vi "OCV Histogram gRPC.vi"() -> (1 "mean values of channels":dbl[](array[numeric]), 2 "std dev":dbl, 3 "range":dbl)   [LabVIEW 2019] (continued)
"battery22voltage"=0.0, "battery23voltage"=0.0, "battery24voltage"=0.0, "ErrorOutData"={"ErrorCode"=0, "ErrorMessage"=""}}, {"battery1voltage"=3.4816399, "battery2voltage"=3.483045, "battery3voltage"=3.4783711, "battery4voltage"=3.482368, "battery5voltage"=3.4843976, "battery6voltage"=0.0, "battery7voltage"=0.0, "battery8voltage"=0.0, "battery9voltage"=0.0, "battery10voltage"=0.0, "battery11voltage"=0.0, "battery12voltage"=0.0, "battery13voltage"=0.0, "battery14voltage"=0.0, "battery15voltage"=0.0, "battery16voltage"=0.0, "battery17voltage"=0.0, "battery18voltage"=0.0, "battery19voltage"=0.0, "battery20voltage"=0.0, "battery21voltage"=0.0, "battery22voltage"=0.0, "battery23voltage"=0.0, "battery24voltage"=0.0, "ErrorOutData"={"ErrorCode"=0, "ErrorMessage"=""}}, {"battery1voltage"=3.4816442, "battery2voltage"=3.4830372, "battery3voltage"=3.4783738, "battery4voltage"=3.482372, "battery5voltage"=3.4844053, "battery6voltage"=0.0, "battery7voltage"=0.0, "battery8voltage"=0.0, "battery9voltage"=0.0, "battery10voltage"=0.0, "battery11voltage"=0.0, "battery12voltage"=0.0, "battery13voltage"=0.0, "battery14voltage"=0.0, "battery15voltage"=0.0, "battery16voltage"=0.0, "battery17voltage"=0.0, "battery18voltage"=0.0, "battery19voltage"=0.0, "battery20voltage"=0.0, "battery21voltage"=0.0, "battery22voltage"=0.0, "battery23voltage"=0.0, "battery24voltage"=0.0, "ErrorOutData"={"ErrorCode"=0, "ErrorMessage"=""}}, {"battery1voltage"=3.4816413, "battery2voltage"=3.4830437, "battery3voltage"=3.4783747, "battery4voltage"=3.482368, "battery5voltage"=3.4843984, "battery6voltage"=0.0, "battery7voltage"=0.0, "battery8voltage"=0.0, "battery9voltage"=0.0, "battery10voltage"=0.0, "battery11voltage"=0.0, "battery12voltage"=0.0, "battery13voltage"=0.0, "battery14voltage"=0.0, "battery15voltage"=0.0, "battery16voltage"=0.0, "battery17voltage"=0.0, "battery18voltage"=0.0, "battery19voltage"=0.0, "battery20voltage"=0.0, "battery21voltage"=0.0, "battery22voltage"=0.0, "battery23voltage"=0.0, "battery24voltage"=0.0, "ErrorOutData"={"ErrorCode"=0, "ErrorMessage"=""}}, {"battery1voltage"=3.481636, "battery2voltage"=3.4830418, "battery3voltage"=3.4783738, "battery4voltage"=3.482369, "battery5voltage"=3.4844093, "battery6voltage"=0.0, "battery7voltage"=0.0, "battery8voltage"=0.0, "battery9voltage"=0.0, "battery10voltage"=0.0, "battery11voltage"=0.0, "battery12voltage"=0.0, "battery13voltage"=0.0, "battery14voltage"=0.0, "battery15voltage"=0.0, "battery16voltage"=0.0, "battery17voltage"=0.0, "battery18voltage"=0.0, "battery19voltage"=0.0, "battery20voltage"=0.0, "battery21voltage"=0.0, "battery22voltage"=0.0, "battery23voltage"=0.0, "battery24voltage"=0.0, "ErrorOutData"={"ErrorCode"=0, "ErrorMessage"=""}}, {"battery1voltage"=3.4816372, "battery2voltage"=3.4830408, "battery3voltage"=3.4783714, "battery4voltage"=3.4823658, "battery5voltage"=3.4844065, "battery6voltage"=0.0, "battery7voltage"=0.0, "battery8voltage"=0.0, "battery9voltage"=0.0, "battery10voltage"=0.0, "battery11voltage"=0.0, "battery12voltage"=0.0, "battery13voltage"=0.0, "battery14voltage"=0.0, "battery15voltage"=0.0, "battery16voltage"=0.0, "battery17voltage"=0.0, "battery18voltage"=0.0, "battery19voltage"=0.0, "battery20voltage"=0.0, "battery21voltage"=0.0, "battery22voltage"=0.0, "battery23voltage"=0.0, "battery24voltage"=0.0, "ErrorOutData"={"ErrorCode"=0, "ErrorMessage"=""}}, {"battery1voltage"=3.4816327, "battery2voltage"=3.4830406, "battery3voltage"=3.47837, "battery4voltage"=3.48237, "battery5voltage"=3.4844074, "battery6voltage"=0.0, "battery7voltage"=0.0, "battery8voltage"=0.0, "battery9voltage"=0.0, "battery10voltage"=0.0, "battery11voltage"=0.0, "battery12voltage"=0.0, "battery13voltage"=0.0, "battery14voltage"=0.0, "battery15voltage"=0.0, "battery16voltage"=0.0, "battery17voltage"=0.0, "battery18voltage"=0.0, "battery19voltage"=0.0, "battery20voltage"=0.0, "battery21voltage"=0.0, "battery22voltage"=0.0, "battery23voltage"=0.0, "battery24voltage"=0.0, "ErrorOutData"={"ErrorCode"=0, "ErrorMessage"=""}}, {"battery1voltage"=3.4816341, "battery2voltage"=3.4830384, "battery3voltage"=3.4783652, "battery4voltage"=3.4823718, "battery5voltage"=3.4844053, "battery6voltage"=0.0, "battery7voltage"=0.0, "battery8voltage"=0.0, "battery9voltage"=0.0, "battery10voltage"=0.0, "battery11voltage"=0.0, "battery12voltage"=0.0, "battery13voltage"=0.0, "battery14voltage"=0.0, "battery15voltage"=0.0, "battery16voltage"=0.0, "battery17voltage"=0.0, "battery18voltage"=0.0, "battery19voltage"=0.0, "battery20voltage"=0.0, "battery21voltage"=0.0, "battery22voltage"=0.0, "battery23voltage"=0.0, "battery24voltage"=0.0, "ErrorOutData"={"ErrorCode"=0, "ErrorMessage"=""}}, {"battery1voltage"=3.4816403, "battery2voltage"=3.4830394, "battery3voltage"=3.4783738, "battery4voltage"=3.482369, "battery5voltage"=3.4843953, "battery6voltage"=0.0, "battery7voltage"=0.0, "battery8voltage"=0.0, "battery9voltage"=0.0, "battery10voltage"=0.0, "battery11voltage"=0.0, "battery12voltage"=0.0, "battery13voltage"=0.0, "battery14voltage"=0.0, "battery15voltage"=0.0, "battery16voltage"=0.0, "battery17voltage"=0.0, "battery18voltage"=0.0, "battery19voltage"=0.0, "battery20voltage"=0.0, "battery21voltage"=0.0, "battery22voltage"=0.0, "battery23voltage"=0.0, "battery24voltage"=0.0, "ErrorOutData"={"ErrorCode"=0, "ErrorMessage"=""}}, {"battery1voltage"=3.4816394, "battery2voltage"=3.4830453, "battery3voltage"=3.4783702, "battery4voltage"=3.4823678, "battery5voltage"=3.4844062, "battery6voltage"=0.0, "battery7voltage"=0.0, "battery8voltage"=0.0, "battery9voltage"=0.0, "battery10voltage"=0.0, "battery11voltage"=0.0, "battery12voltage"=0.0, "battery13voltage"=0.0, "battery14voltage"=0.0, "battery15voltage"=0.0, "battery16voltage"=0.0, "battery17voltage"=0.0, "battery18voltage"=0.0, "battery19voltage"=0.0, "battery20voltage"=0.0, "battery21voltage"=0.0, "battery22voltage"=0.0, "battery23voltage"=0.0, "battery24voltage"=0.0, "ErrorOutData"={"ErrorCode"=0, "ErrorMessage"=""}}, {"battery1voltage"=3.4816413, "battery2voltage"=3.4830458, "battery3voltage"=3.478368, "battery4voltage"=3.482369, "battery5voltage"=3.4844098, "battery6voltage"=0.0, "battery7voltage"=0.0, "battery8voltage"=0.0, "battery9voltage"=0.0, "battery10voltage"=0.0, "battery11voltage"=0.0, "battery12voltage"=0.0, "battery13voltage"=0.0, "battery14voltage"=0.0, "battery15voltage"=0.0, "battery16voltage"=0.0, "battery17voltage"=0.0, "battery18voltage"=0.0, "battery19voltage"=0.0, "battery20voltage"=0.0, "battery21voltage"=0.0, "battery22voltage"=0.0, "battery23voltage"=0.0, "battery24voltage"=0.0, "ErrorOutData"={"ErrorCode"=0, "ErrorMessage"=""}}, {"battery1voltage"=3.4816415, "battery2voltage"=3.4830437, "battery3voltage"=3.4783766, "battery4voltage"=3.4823713, "battery5voltage"=3.4844012, "battery6voltage"=0.0, "battery7voltage"=0.0, "battery8voltage"=0.0, "battery9voltage"=0.0, "battery10voltage"=0.0, "battery11voltage"=0.0, "battery12voltage"=0.0, "battery13voltage"=0.0, "battery14voltage"=0.0, "battery15voltage"=0.0, "battery16voltage"=0.0, "battery17voltage"=0.0, "battery18voltage"=0.0, "battery19voltage"=0.0, "battery20voltage"=0.0, "battery21voltage"=0.0, "battery22voltage"=0.0, "battery23voltage"=0.0, "battery24voltage"=0.0, "ErrorOutData"={"ErrorCode"=0, "ErrorMessage"=""}}, {"battery1voltage"=3.4816406, "battery2voltage"=3.4830434, "battery3voltage"=3.4783766, "battery4voltage"=3.4823692, "battery5voltage"=3.4844048, "battery6voltage"=0.0, "battery7voltage"=0.0, "battery8voltage"=0.0, "battery9voltage"=0.0, "battery10voltage"=0.0, "battery11voltage"=0.0, "battery12voltage"=0.0, "battery13voltage"=0.0, "battery14voltage"=0.0, "battery15voltage"=0.0, "battery16voltage"=0.0, "battery17voltage"=0.0, "battery18voltage"=0.0, "battery19voltage"=0.0, "battery20voltage"=0.0, "battery21voltage"=0.0, "battery22voltage"=0.0, "battery23voltage"=0.0, "battery24voltage"=0.0, "ErrorOutData"={"ErrorCode"=0, "ErrorMessage"=""}}, {"battery1voltage"=3.481637, "battery2voltage"=3.4830406, "battery3voltage"=3.478371, "battery4voltage"=3.4823666, "battery5voltage"=3.4844093, "battery6voltage"=0.0, "battery7voltage"=0.0, "battery8voltage"=0.0, "battery9voltage"=0.0, "battery10voltage"=0.0, "battery11voltage"=0.0, "battery12voltage"=0.0, "battery13voltage"=0.0, "battery14voltage"=0.0, "battery15voltage"=0.0, "battery16voltage"=0.0, "battery17voltage"=0.0, "battery18voltage"=0.0, "battery19voltage"=0.0, "battery20voltage"=0.0, "battery21voltage"=0.0, "battery22voltage"=0.0, "battery23voltage"=0.0, "battery24voltage"=0.0, "ErrorOutData"={"ErrorCode"=0, "ErrorMessage"=""}}, {"battery1voltage"=3.4816372, "battery2voltage"=3.4830427, "battery3voltage"=3.4783697, "battery4voltage"=3.4823666, "battery5voltage"=3.4844093, "battery6voltage"=0.0, "battery7voltage"=0.0, "battery8voltage"=0.0, "battery9voltage"=0.0, "battery10voltage"=0.0, "battery11voltage"=0.0, "battery12voltage"=0.0, "battery13voltage"=0.0, "battery14voltage"=0.0, "battery15voltage"=0.0, "battery16voltage"=0.0, "battery17voltage"=0.0, "battery18voltage"=0.0, "battery19voltage"=0.0, "battery20voltage"=0.0, "battery21voltage"=0.0, "battery22voltage"=0.0, "battery23voltage"=0.0, "battery24voltage"=0.0, "ErrorOutData"={"ErrorCode"=0, "ErrorMessage"=""}}, {"battery1voltage"=3.4816396, "battery2voltage"=3.483044, "battery3voltage"=3.4783752, "battery4voltage"=3.4823713, "battery5voltage"=3.4844036, "battery6voltage"=0.0, "battery7voltage"=0.0, "battery8voltage"=0.0, "battery9voltage"=0.0, "battery10voltage"=0.0, "battery11voltage"=0.0, "battery12voltage"=0.0, "battery13voltage"=0.0, "battery14voltage"=0.0, "battery15voltage"=0.0, "battery16voltage"=0.0, "battery17voltage"=0.0, "battery18voltage"=0.0, "battery19voltage"=0.0, "battery20voltage"=0.0, "battery21voltage"=0.0, "battery22voltage"=0.0, "battery23voltage"=0.0, "battery24voltage"=0.0, "ErrorOutData"={"ErrorCode"=0, "ErrorMessage"=""}}, {"battery1voltage"=3.4816391, "battery2voltage"=3.4830427, "battery3voltage"=3.478371, "battery4voltage"=3.482368, "battery5voltage"=3.4844048, "battery6voltage"=0.0, "battery7voltage"=0.0, "battery8voltage"=0.0, "battery9voltage"=0.0, "battery10voltage"=0.0, "battery11voltage"=0.0, "battery12voltage"=0.0, "battery13voltage"=0.0, "battery14voltage"=0.0, "battery15voltage"=0.0, "battery16voltage"=0.0, "battery17voltage"=0.0, "battery18voltage"=0.0, "battery19voltage"=0.0, "battery20voltage"=0.0, "battery21voltage"=0.0, "battery22voltage"=0.0, "battery23voltage"=0.0, "battery24voltage"=0.0, "ErrorOutData"={"ErrorCode"=0, "ErrorMessage"=""}}, {"battery1voltage"=3.481643, "battery2voltage"=3.4830446, "battery3voltage"=3.4783757, "battery4voltage"=3.482366, "battery5voltage"=3.4843988, "battery6voltage"=0.0, "battery7voltage"=0.0, "battery8voltage"=0.0, "battery9voltage"=0.0, "battery10voltage"=0.0, "battery11voltage"=0.0, "battery12voltage"=0.0, "battery13voltage"=0.0, "battery14voltage"=0.0, "battery15voltage"=0.0, "battery16voltage"=0.0, "battery17voltage"=0.0, "battery18voltage"=0.0, "battery19voltage"=0.0, "battery20voltage"=0.0, "battery21voltage"=0.0, "battery22voltage"=0.0, "battery23voltage"=0.0, "battery24voltage"=0.0, "ErrorOutData"={"ErrorCode"=0, "ErrorMessage"=""}}, {"battery1voltage"=3.4816375, "battery2voltage"=3.4830432, "battery3voltage"=3.47837, "battery4voltage"=3.482367, "battery5voltage"=3.4844115, "battery6voltage"=0.0, "battery7voltage"=0.0, "battery8voltage"=0.0, "battery9voltage"=0.0, "battery10voltage"=0.0, "battery11voltage"=0.0, "battery12voltage"=0.0, "battery13voltage"=0.0, "battery14voltage"=0.0, "battery15voltage"=0.0, "battery16voltage"=0.0, "battery17voltage"=0.0, "battery18voltage"=0.0, "battery19voltage"=0.0, "battery20voltage"=0.0, "battery21voltage"=0.0, "battery22voltage"=0.0, "battery23voltage"=0.0, "battery24voltage"=0.0, "ErrorOutData"={"ErrorCode"=0, "ErrorMessage"=""}}, {"battery1voltage"=3.4816341, "battery2voltage"=3.4830444, "battery3voltage"=3.4783678, "battery4voltage"=3.48237, "battery5voltage"=3.4844046, "battery6voltage"=0.0, "battery7voltage"=0.0, "battery8voltage"=0.0, "battery9voltage"=0.0, "battery10voltage"=0.0, "battery11voltage"=0.0, "battery12voltage"=0.0, "battery13voltage"=0.0, "battery14voltage"=0.0, "battery15voltage"=0.0, "battery16voltage"=0.0, "battery17voltage"=0.0, "battery18voltage"=0.0, "battery19voltage"=0.0, "battery20voltage"=0.0, "battery21voltage"=0.0, "battery22voltage"=0.0, "battery23voltage"=0.0, "battery24voltage"=0.0, "ErrorOutData"={"ErrorCode"=0, "ErrorMessage"=""}}, {"battery1voltage"=3.4816446, "battery2voltage"=3.4830422, "battery3voltage"=3.4783723, "battery4voltage"=3.4823694, "battery5voltage"=3.4844015, "battery6voltage"=0.0, "battery7voltage"=0.0, "battery8voltage"=0.0, "battery9voltage"=0.0, "battery10voltage"=0.0, "battery11voltage"=0.0, "battery12voltage"=0.0, "battery13voltage"=0.0, "battery14voltage"=0.0, "battery15voltage"=0.0, "battery16voltage"=0.0, "battery17voltage"=0.0, "battery18voltage"=0.0, "battery19voltage"=0.0, "battery20voltage"=0.0, "battery21voltage"=0.0, "battery22voltage"=0.0, "battery23voltage"=0.0, "battery24voltage"=0.0, "ErrorOutData"={"ErrorCode"=0, "ErrorMessage"=""}}, {"battery1voltage"=3.4816337, "battery2voltage"=3.483039, "battery3voltage"=3.4783669, "battery4voltage"=3.4823694, "battery5voltage"=3.4844108, "battery6voltage"=0.0, "battery7voltage"=0.0, "battery8voltage"=0.0, "battery9voltage"=0.0, "battery10voltage"=0.0, "battery11voltage"=0.0, "battery12voltage"=0.0, "battery13voltage"=0.0, "battery14voltage"=0.0, "battery15voltage"=0.0, "battery16voltage"=0.0, "battery17voltage"=0.0, "battery18voltage"=0.0, "battery19voltage"=0.0, "battery20voltage"=0.0, "battery21voltage"=0.0, "battery22voltage"=0.0, "battery23voltage"=0.0, "battery24voltage"=0.0, "ErrorOutData"={"ErrorCode"=0, "ErrorMessage"=""}}, {"battery1voltage"=3.4816325, "battery2voltage"=3.4830413, "battery3voltage"=3.4783652, "battery4voltage"=3.4823673, "battery5voltage"=3.4844015, "battery6voltage"=0.0, "battery7voltage"=0.0, "battery8voltage"=0.0, "battery9voltage"=0.0, "battery10voltage"=0.0, "battery11voltage"=0.0, "battery12voltage"=0.0, "battery13voltage"=0.0, "battery14voltage"=0.0, "battery15voltage"=0.0, "battery16voltage"=0.0, "battery17voltage"=0.0, "battery18voltage"=0.0, "battery19voltage"=0.0, "battery20voltage"=0.0, "battery21voltage"=0.0, "battery22voltage"=0.0, "battery23voltage"=0.0, "battery24voltage"=0.0, "ErrorOutData"={"ErrorCode"=0, "ErrorMessage"=""}}, {"battery1voltage"=3.4816356, "battery2voltage"=3.483046, "battery3voltage"=3.478368, "battery4voltage"=3.482366, "battery5voltage"=3.4844065, "battery6voltage"=0.0, "battery7voltage"=0.0, "battery8voltage"=0.0, "battery9voltage"=0.0, "battery10voltage"=0.0, "battery11voltage"=0.0, "battery12voltage"=0.0, "battery13voltage"=0.0, "battery14voltage"=0.0, "battery15voltage"=0.0, "battery16voltage"=0.0, "battery17voltage"=0.0, "battery18voltage"=0.0, "battery19voltage"=0.0, "battery20voltage"=0.0, "battery21voltage"=0.0, "battery22voltage"=0.0, "battery23voltage"=0.0, "battery24voltage"=0.0, "ErrorOutData"={"ErrorCode"=0, "ErrorMessage"=""}}, {"battery1voltage"=3.4816365, "battery2voltage"=3.4830458, "battery3voltage"=3.4783702, "battery4voltage"=3.4823682, "battery5voltage"=3.484401, "battery6voltage"=0.0, "battery7voltage"=0.0, "battery8voltage"=0.0, "battery9voltage"=0.0, "battery10voltage"=0.0, "battery11voltage"=0.0, "battery12voltage"=0.0, "battery13voltage"=0.0, "battery14voltage"=0.0, "battery15voltage"=0.0, "battery16voltage"=0.0, "battery17voltage"=0.0, "battery18voltage"=0.0, "battery19voltage"=0.0, "battery20voltage"=0.0, "battery21voltage"=0.0, "battery22voltage"=0.0, "battery23voltage"=0.0, "battery24voltage"=0.0, "ErrorOutData"={"ErrorCode"=0, "ErrorMessage"=""}}, {"battery1voltage"=3.4816322, "battery2voltage"=3.4830444, "battery3voltage"=3.4783752, "battery4voltage"=3.4823666, "battery5voltage"=3.4844022, "battery6voltage"=0.0, "battery7voltage"=0.0, "battery8voltage"=0.0, "battery9voltage"=0.0, "battery10voltage"=0.0, "battery11voltage"=0.0, "battery12voltage"=0.0, "battery13voltage"=0.0, "battery14voltage"=0.0, "battery15voltage"=0.0, "battery16voltage"=0.0, "battery17voltage"=0.0, "battery18voltage"=0.0, "battery19voltage"=0.0, "battery20voltage"=0.0, "battery21voltage"=0.0, "battery22voltage"=0.0, "battery23voltage"=0.0, "battery24voltage"=0.0, "ErrorOutData"={"ErrorCode"=0, "ErrorMessage"=""}}, {"battery1voltage"=3.4816391, "battery2voltage"=3.4830413, "battery3voltage"=3.4783728, "battery4voltage"=3.4823685, "battery5voltage"=3.4844005, "battery6voltage"=0.0, "battery7voltage"=0.0, "battery8voltage"=0.0, "battery9voltage"=0.0, "battery10voltage"=0.0, "battery11voltage"=0.0, "battery12voltage"=0.0, "battery13voltage"=0.0, "battery14voltage"=0.0, "battery15voltage"=0.0, "battery16voltage"=0.0, "battery17voltage"=0.0, "battery18voltage"=0.0, "battery19voltage"=0.0, "battery20voltage"=0.0, "battery21voltage"=0.0, "battery22voltage"=0.0, "battery23voltage"=0.0, "battery24voltage"=0.0, "ErrorOutData"={"ErrorCode"=0, "ErrorMessage"=""}}, {"battery1voltage"=3.481637, "battery2voltage"=3.4830399, "battery3voltage"=3.4783745, "battery4voltage"=3.482366, "battery5voltage"=3.4844046, "battery6voltage"=0.0, "battery7voltage"=0.0, "battery8voltage"=0.0, "battery9voltage"=0.0, "battery10voltage"=0.0, "battery11voltage"=0.0, "battery12voltage"=0.0, "battery13voltage"=0.0, "battery14voltage"=0.0, "battery15voltage"=0.0, "battery16voltage"=0.0, "battery17voltage"=0.0, "battery18voltage"=0.0, "battery19voltage"=0.0, "battery20voltage"=0.0, "battery21voltage"=0.0, "battery22voltage"=0.0, "battery23voltage"=0.0, "battery24voltage"=0.0, "ErrorOutData"={"ErrorCode"=0, "ErrorMessage"=""}}, {"battery1voltage"=3.4816382, "battery2voltage"=3.4830427, "battery3voltage"=3.4783697, "battery4voltage"=3.48237, "battery5voltage"=3.4844015, "battery6voltage"=0.0, "battery7voltage"=0.0, "battery8voltage"=0.0, "battery9voltage"=0.0, "battery10voltage"=0.0, "battery11voltage"=0.0, "battery12voltage"=0.0, "battery13voltage"=0.0, "battery14voltage"=0.0, "battery15voltage"=0.0, "battery16voltage"=0.0, "battery17voltage"=0.0, "battery18voltage"=0.0, "battery19voltage"=0.0, "battery20voltage"=0.0, "battery21voltage"=0.0, "battery22voltage"=0.0, "battery23voltage"=0.0, "battery24voltage"=0.0, "ErrorOutData"={"ErrorCode"=0, "ErrorMessage"=""}}, {"battery1voltage"=3.4816358, "battery2voltage"=3.4830434, "battery3voltage"=3.4783742, "battery4voltage"=3.4823682, "battery5voltage"=3.4844017, "battery6voltage"=0.0, "battery7voltage"=0.0, "battery8voltage"=0.0, "battery9voltage"=0.0, "battery10voltage"=0.0, "battery11voltage"=0.0, "battery12voltage"=0.0, "battery13voltage"=0.0, "battery14voltage"=0.0, "battery15voltage"=0.0, "battery16voltage"=0.0, "battery17voltage"=0.0, "battery18voltage"=0.0, "battery19voltage"=0.0, "battery20voltage"=0.0, "battery21voltage"=0.0, "battery22voltage"=0.0, "battery23voltage"=0.0, "battery24voltage"=0.0, "ErrorOutData"={"ErrorCode"=0, "ErrorMessage"=""}}, {"battery1voltage"=3.4816394, "battery2voltage"=3.483044, "battery3voltage"=3.4783754, "battery4voltage"=3.4823692, "battery5voltage"=3.4844005, "battery6voltage"=0.0, "battery7voltage"=0.0, "battery8voltage"=0.0, "battery9voltage"=0.0, "battery10voltage"=0.0, "battery11voltage"=0.0, "battery12voltage"=0.0, "battery13voltage"=0.0, "battery14voltage"=0.0, "battery15voltage"=0.0, "battery16voltage"=0.0, "battery17voltage"=0.0, "battery18voltage"=0.0, "battery19voltage"=0.0, "battery20voltage"=0.0, "battery21voltage"=0.0, "battery22voltage"=0.0, "battery23voltage"=0.0, "battery24voltage"=0.0, "ErrorOutData"={"ErrorCode"=0, "ErrorMessage"=""}}, {"battery1voltage"=3.481634, "battery2voltage"=3.4830408, "battery3voltage"=3.4783669, "battery4voltage"=3.4823651, "battery5voltage"=3.4844038, "battery6voltage"=0.0, "battery7voltage"=0.0, "battery8voltage"=0.0, "battery9voltage"=0.0, "battery10voltage"=0.0, "battery11voltage"=0.0, "battery12voltage"=0.0, "battery13voltage"=0.0, "battery14voltage"=0.0, "battery15voltage"=0.0, "battery16voltage"=0.0, "battery17voltage"=0.0, "battery18voltage"=0.0, "battery19voltage"=0.0, "battery20voltage"=0.0, "battery21voltage"=0.0, "battery22voltage"=0.0, "battery23voltage"=0.0, "battery24voltage"=0.0, "ErrorOutData"={"ErrorCode"=0, "ErrorMessage"=""}}, {"battery1voltage"=3.4816377, "battery2voltage"=3.4830425, "battery3voltage"=3.4783716, "battery4voltage"=3.482369, "battery5voltage"=3.484401, "battery6voltage"=0.0, "battery7voltage"=0.0, "battery8voltage"=0.0, "battery9voltage"=0.0, "battery10voltage"=0.0, "battery11voltage"=0.0, "battery12voltage"=0.0, "battery13voltage"=0.0, "battery14voltage"=0.0, "battery15voltage"=0.0, "battery16voltage"=0.0, "battery17voltage"=0.0, "battery18voltage"=0.0, "battery19voltage"=0.0, "battery20voltage"=0.0, "battery21voltage"=0.0, "battery22voltage"=0.0, "battery23voltage"=0.0, "battery24voltage"=0.0, "ErrorOutData"={"ErrorCode"=0, "ErrorMessage"=""}}, {"battery1voltage"=3.481638, "battery2voltage"=3.483039, "battery3voltage"=3.4783654, "battery4voltage"=3.48237, "battery5voltage"=3.4844065, "battery6voltage"=0.0, "battery7voltage"=0.0, "battery8voltage"=0.0, "battery9voltage"=0.0, "battery10voltage"=0.0, "battery11voltage"=0.0, "battery12voltage"=0.0, "battery13voltage"=0.0, "battery14voltage"=0.0, "battery15voltage"=0.0, "battery16voltage"=0.0, "battery17voltage"=0.0, "battery18voltage"=0.0, "battery19voltage"=0.0, "battery20voltage"=0.0, "battery21voltage"=0.0, "battery22voltage"=0.0, "battery23voltage"=0.0, "battery24voltage"=0.0, "ErrorOutData"={"ErrorCode"=0, "ErrorMessage"=""}}, {"battery1voltage"=3.4816375, "battery2voltage"=3.4830475, "battery3voltage"=3.4783783, "battery4voltage"=3.4823647, "battery5voltage"=3.4844038, "battery6voltage"=0.0, "battery7voltage"=0.0, "battery8voltage"=0.0, "battery9voltage"=0.0, "battery10voltage"=0.0, "battery11voltage"=0.0, "battery12voltage"=0.0, "battery13voltage"=0.0, "battery14voltage"=0.0, "battery15voltage"=0.0, "battery16voltage"=0.0, "battery17voltage"=0.0, "battery18voltage"=0.0, "battery19voltage"=0.0, "battery20voltage"=0.0, "battery21voltage"=0.0, "battery22voltage"=0.0, "battery23voltage"=0.0, "battery24voltage"=0.0, "ErrorOutData"={"ErrorCode"=0, "ErrorMessage"=""}}, {"battery1voltage"=3.4816403, "battery2voltage"=3.4830472, "battery3voltage"=3.4783723, "battery4voltage"=3.4823694, "battery5voltage"=3.4843976, "battery6voltage"=0.0, "battery7voltage"=0.0, "battery8voltage"=0.0, "battery9voltage"=0.0, "battery10voltage"=0.0, "battery11voltage"=0.0, "battery12voltage"=0.0, "battery13voltage"=0.0, "battery14voltage"=0.0, "battery15voltage"=0.0, "battery16voltage"=0.0, "battery17voltage"=0.0, "battery18voltage"=0.0, "battery19voltage"=0.0, "battery20voltage"=0.0, "battery21voltage"=0.0, "battery22voltage"=0.0, "battery23voltage"=0.0, "battery24voltage"=0.0, "ErrorOutData"={"ErrorCode"=0, "ErrorMessage"=""}}, {"battery1voltage"=3.4816413, "battery2voltage"=3.4830482, "battery3voltage"=3.4783695, "battery4voltage"=3.482367, "battery5voltage"=3.4844043, "battery6voltage"=0.0, "battery7voltage"=0.0, "battery8voltage"=0.0, "battery9voltage"=0.0, "battery10voltage"=0.0, "battery11voltage"=0.0, "battery12voltage"=0.0, "battery13voltage"=0.0, "battery14voltage"=0.0, "battery15voltage"=0.0, "battery16voltage"=0.0, "battery17voltage"=0.0, "battery18voltage"=0.0, "battery19voltage"=0.0, "battery20voltage"=0.0, "battery21voltage"=0.0, "battery22voltage"=0.0, "battery23voltage"=0.0, "battery24voltage"=0.0, "ErrorOutData"={"ErrorCode"=0, "ErrorMessage"=""}}, {"battery1voltage"=3.4816382, "battery2voltage"=3.4830446, "battery3voltage"=3.4783735, "battery4voltage"=3.4823701, "battery5voltage"=3.4843962, "battery6voltage"=0.0, "battery7voltage"=0.0, "battery8voltage"=0.0, "battery9voltage"=0.0, "battery10voltage"=0.0, "battery11voltage"=0.0, "battery12voltage"=0.0, "battery13voltage"=0.0, "battery14voltage"=0.0, "battery15voltage"=0.0, "battery16voltage"=0.0, "battery17voltage"=0.0, "battery18voltage"=0.0, "battery19voltage"=0.0, "battery20voltage"=0.0, "battery21voltage"=0.0, "battery22voltage"=0.0, "battery23voltage"=0.0, "battery24voltage"=0.0, "ErrorOutData"={"ErrorCode"=0, "ErrorMessage"=""}}, {"battery1voltage"=3.481636, "battery2voltage"=3.4830408, "battery3voltage"=3.4783683, "battery4voltage"=3.482367, "battery5voltage"=3.484406, "battery6voltage"=0.0, "battery7voltage"=0.0, "battery8voltage"=0.0, "battery9voltage"=0.0, "battery10voltage"=0.0, "battery11voltage"=0.0, "battery12voltage"=0.0, "battery13voltage"=0.0, "battery14voltage"=0.0, "battery15voltage"=0.0, "battery16voltage"=0.0, "battery17voltage"=0.0, "battery18voltage"=0.0, "battery19voltage"=0.0, "battery20voltage"=0.0, "battery21voltage"=0.0, "battery22voltage"=0.0, "battery23voltage"=0.0, "battery24voltage"=0.0, "ErrorOutData"={"ErrorCode"=0, "ErrorMessage"=""}}, {"battery1voltage"=3.4816418, "battery2voltage"=3.4830418, "battery3voltage"=3.4783669, "battery4voltage"=3.482368, "battery5voltage"=3.484411, "battery6voltage"=0.0, "battery7voltage"=0.0, "battery8voltage"=0.0, "battery9voltage"=0.0, "battery10voltage"=0.0, "battery11voltage"=0.0, "battery12voltage"=0.0, "battery13voltage"=0.0, "battery14voltage"=0.0, "battery15voltage"=0.0, "battery16voltage"=0.0, "battery17voltage"=0.0, "battery18voltage"=0.0, "battery19voltage"=0.0, "battery20voltage"=0.0, "battery21voltage"=0.0, "battery22voltage"=0.0, "battery23voltage"=0.0, "battery24voltage"=0.0, "ErrorOutData"={"ErrorCode"=0, "ErrorMessage"=""}}, {"battery1voltage"=3.4816382, "battery2voltage"=3.483042, "battery3voltage"=3.4783723, "battery4voltage"=3.4823678, "battery5voltage"=3.4844053, "battery6voltage"=0.0, "battery7voltage"=0.0, "battery8voltage"=0.0, "battery9voltage"=0.0, "battery10voltage"=0.0, "battery11voltage"=0.0, "battery12voltage"=0.0, "battery13voltage"=0.0, "battery14voltage"=0.0, "battery15voltage"=0.0, "battery16voltage"=0.0, "battery17voltage"=0.0, "battery18voltage"=0.0, "battery19voltage"=0.0, "battery20voltage"=0.0, "battery21voltage"=0.0, "battery22voltage"=0.0, "battery23voltage"=0.0, "battery24voltage"=0.0, "ErrorOutData"={"ErrorCode"=0, "ErrorMessage"=""}}, {"battery1voltage"=3.4816322, "battery2voltage"=3.4830375, "battery3voltage"=3.478369, "battery4voltage"=3.4823651, "battery5voltage"=3.484405, "battery6voltage"=0.0, "battery7voltage"=0.0, "battery8voltage"=0.0, "battery9voltage"=0.0, "battery10voltage"=0.0, "battery11voltage"=0.0, "battery12voltage"=0.0, "battery13voltage"=0.0, "battery14voltage"=0.0, "battery15voltage"=0.0, "battery16voltage"=0.0, "battery17voltage"=0.0, "battery18voltage"=0.0, "battery19voltage"=0.0, "battery20voltage"=0.0, "battery21voltage"=0.0, "battery22voltage"=0.0, "battery23voltage"=0.0, "battery24voltage"=0.0, "ErrorOutData"={"ErrorCode"=0, "ErrorMessage"=""}}, {"battery1voltage"=3.4816375, "battery2voltage"=3.4830382, "battery3voltage"=3.478371, "battery4voltage"=3.4823635, "battery5voltage"=3.4844062, "battery6voltage"=0.0, "battery7voltage"=0.0, "battery8voltage"=0.0, "battery9voltage"=0.0, "battery10voltage"=0.0, "battery11voltage"=0.0, "battery12voltage"=0.0, "battery13voltage"=0.0, "battery14voltage"=0.0, "battery15voltage"=0.0, "battery16voltage"=0.0, "battery17voltage"=0.0, "battery18voltage"=0.0, "battery19voltage"=0.0, "battery20voltage"=0.0, "battery21voltage"=0.0, "battery22voltage"=0.0, "battery23voltage"=0.0, "battery24voltage"=0.0, "ErrorOutData"={"ErrorCode"=0, "ErrorMessage"=""}}, {"battery1voltage"=3.4816356, "battery2voltage"=3.4830391, "battery3voltage"=3.4783695, "battery4voltage"=3.482366, "battery5voltage"=3.4844058, "battery6voltage"=0.0, "battery7voltage"=0.0, "battery8voltage"=0.0, "battery9voltage"=0.0, "battery10voltage"=0.0, "battery11voltage"=0.0, "battery12voltage"=0.0, "battery13voltage"=0.0, "battery14voltage"=0.0, "battery15voltage"=0.0, "battery16voltage"=0.0, "battery17voltage"=0.0, "battery18voltage"=0.0, "battery19voltage"=0.0, "battery20voltage"=0.0, "battery21voltage"=0.0, "battery22voltage"=0.0, "battery23voltage"=0.0, "battery24voltage"=0.0, "ErrorOutData"={"ErrorCode"=0, "ErrorMessage"=""}}, {"battery1voltage"=3.481642, "battery2voltage"=3.483044, "battery3voltage"=3.4783707, "battery4voltage"=3.482366, "battery5voltage"=3.4844027, "battery6voltage"=0.0, "battery7voltage"=0.0, "battery8voltage"=0.0, "battery9voltage"=0.0, "battery10voltage"=0.0, "battery11voltage"=0.0, "battery12voltage"=0.0, "battery13voltage"=0.0, "battery14voltage"=0.0, "battery15voltage"=0.0, "battery16voltage"=0.0, "battery17voltage"=0.0, "battery18voltage"=0.0, "battery19voltage"=0.0, "battery20voltage"=0.0, "battery21voltage"=0.0, "battery22voltage"=0.0, "battery23voltage"=0.0, "battery24voltage"=0.0, "ErrorOutData"={"ErrorCode"=0, "ErrorMessage"=""}}, {"battery1voltage"=3.4816384, "battery2voltage"=3.483043, "battery3voltage"=3.4783728, "battery4voltage"=3.4823685, "battery5voltage"=3.4844081, "battery6voltage"=0.0, "battery7voltage"=0.0, "battery8voltage"=0.0, "battery9voltage"=0.0, "battery10voltage"=0.0, "battery11voltage"=0.0, "battery12voltage"=0.0, "battery13voltage"=0.0, "battery14voltage"=0.0, "battery15voltage"=0.0, "battery16voltage"=0.0, "battery17voltage"=0.0, "battery18voltage"=0.0, "battery19voltage"=0.0, "battery20voltage"=0.0, "battery21voltage"=0.0, "battery22voltage"=0.0, "battery23voltage"=0.0, "battery24voltage"=0.0, "ErrorOutData"={"ErrorCode"=0, "ErrorMessage"=""}}, {"battery1voltage"=3.4816382, "battery2voltage"=3.4830403, "battery3voltage"=3.4783695, "battery4voltage"=3.4823694, "battery5voltage"=3.4844038, "battery6voltage"=0.0, "battery7voltage"=0.0, "battery8voltage"=0.0, "battery9voltage"=0.0, "battery10voltage"=0.0, "battery11voltage"=0.0, "battery12voltage"=0.0, "battery13voltage"=0.0, "battery14voltage"=0.0, "battery15voltage"=0.0, "battery16voltage"=0.0, "battery17voltage"=0.0, "battery18voltage"=0.0, "battery19voltage"=0.0, "battery20voltage"=0.0, "battery21voltage"=0.0, "battery22voltage"=0.0, "battery23voltage"=0.0, "battery24voltage"=0.0, "ErrorOutData"={"ErrorCode"=0, "ErrorMessage"=""}}, {"battery1voltage"=3.4816365, "battery2voltage"=3.4830384, "battery3voltage"=3.4783714, "battery4voltage"=3.4823656, "battery5voltage"=3.484406, "battery6voltage"=0.0, "battery7voltage"=0.0, "battery8voltage"=0.0, "battery9voltage"=0.0, "battery10voltage"=0.0, "battery11voltage"=0.0, "battery12voltage"=0.0, "battery13voltage"=0.0, "battery14voltage"=0.0, "battery15voltage"=0.0, "battery16voltage"=0.0, "battery17voltage"=0.0, "battery18voltage"=0.0, "battery19voltage"=0.0, "battery20voltage"=0.0, "battery21voltage"=0.0, "battery22voltage"=0.0, "battery23voltage"=0.0, "battery24voltage"=0.0, "ErrorOutData"={"ErrorCode"=0, "ErrorMessage"=""}}, {"battery1voltage"=3.481637, "battery2voltage"=3.4830413, "battery3voltage"=3.478368, "battery4voltage"=3.4823709, "battery5voltage"=3.4844017, "battery6voltage"=0.0, "battery7voltage"=0.0, "battery8voltage"=0.0, "battery9voltage"=0.0, "battery10voltage"=0.0, "battery11voltage"=0.0, "battery12voltage"=0.0, "battery13voltage"=0.0, "battery14voltage"=0.0, "battery15voltage"=0.0, "battery16voltage"=0.0, "battery17voltage"=0.0, "battery18voltage"=0.0, "battery19voltage"=0.0, "battery20voltage"=0.0, "battery21voltage"=0.0, "battery22voltage"=0.0, "battery23voltage"=0.0, "battery24voltage"=0.0, "ErrorOutData"={"ErrorCode"=0, "ErrorMessage"=""}}, {"battery1voltage"=3.4816353, "battery2voltage"=3.483047, "battery3voltage"=3.4783692, "battery4voltage"=3.4823658, "battery5voltage"=3.4844015, "battery6voltage"=0.0, "battery7voltage"=0.0, "battery8voltage"=0.0, "battery9voltage"=0.0, "battery10voltage"=0.0, "battery11voltage"=0.0, "battery12voltage"=0.0, "battery13voltage"=0.0, "battery14voltage"=0.0, "battery15voltage"=0.0, "battery16voltage"=0.0, "battery17voltage"=0.0, "battery18voltage"=0.0, "battery19voltage"=0.0, "battery20voltage"=0.0, "battery21voltage"=0.0, "battery22voltage"=0.0, "battery23voltage"=0.0, "battery24voltage"=0.0, "ErrorOutData"={"ErrorCode"=0, "ErrorMessage"=""}}, {"battery1voltage"=3.4816394, "battery2voltage"=3.4830372, "battery3voltage"=3.4783678, "battery4voltage"=3.4823673, "battery5voltage"=3.4844034, "battery6voltage"=0.0, "battery7voltage"=0.0, "battery8voltage"=0.0, "battery9voltage"=0.0, "battery10voltage"=0.0, "battery11voltage"=0.0, "battery12voltage"=0.0, "battery13voltage"=0.0, "battery14voltage"=0.0, "battery15voltage"=0.0, "battery16voltage"=0.0, "battery17voltage"=0.0, "battery18voltage"=0.0, "battery19voltage"=0.0, "battery20voltage"=0.0, "battery21voltage"=0.0, "battery22voltage"=0.0, "battery23voltage"=0.0, "battery24voltage"=0.0, "ErrorOutData"={"ErrorCode"=0, "ErrorMessage"=""}}, {"battery1voltage"=3.4816382, "battery2voltage"=3.4830408, "battery3voltage"=3.4783669, "battery4voltage"=3.4823682, "battery5voltage"=3.4844112, "battery6voltage"=0.0, "battery7voltage"=0.0, "battery8voltage"=0.0, "battery9voltage"=0.0, "battery10voltage"=0.0, "battery11voltage"=0.0, "battery12voltage"=0.0, "battery13voltage"=0.0, "battery14voltage"=0.0, "battery15voltage"=0.0, "battery16voltage"=0.0, "battery17voltage"=0.0, "battery18voltage"=0.0, "battery19voltage"=0.0, "battery20voltage"=0.0, "battery21voltage"=0.0, "battery22voltage"=0.0, "battery23voltage"=0.0, "battery24voltage"=0.0, "ErrorOutData"={"ErrorCode"=0, "ErrorMessage"=""}}, {"battery1voltage"=3.4816437, "battery2voltage"=3.483042, "battery3voltage"=3.4783704, "battery4voltage"=3.4823694, "battery5voltage"=3.4844022, "battery6voltage"=0.0, "battery7voltage"=0.0, "battery8voltage"=0.0, "battery9voltage"=0.0, "battery10voltage"=0.0, "battery11voltage"=0.0, "battery12voltage"=0.0, "battery13voltage"=0.0, "battery14voltage"=0.0, "battery15voltage"=0.0, "battery16voltage"=0.0, "battery17voltage"=0.0, "battery18voltage"=0.0, "battery19voltage"=0.0, "battery20voltage"=0.0, "battery21voltage"=0.0, "battery22voltage"=0.0, "battery23voltage"=0.0, "battery24voltage"=0.0, "ErrorOutData"={"ErrorCode"=0, "ErrorMessage"=""}}, {"battery1voltage"=3.4816415, "battery2voltage"=3.483049, "battery3voltage"=3.4783702, "battery4voltage"=3.482367, "battery5voltage"=3.4844034, "battery6voltage"=0.0, "battery7voltage"=0.0, "battery8voltage"=0.0, "battery9voltage"=0.0, "battery10voltage"=0.0, "battery11voltage"=0.0, "battery12voltage"=0.0, "battery13voltage"=0.0, "battery14voltage"=0.0, "battery15voltage"=0.0, "battery16voltage"=0.0, "battery17voltage"=0.0, "battery18voltage"=0.0, "battery19voltage"=0.0, "battery20voltage"=0.0, "battery21voltage"=0.0, "battery22voltage"=0.0, "battery23voltage"=0.0, "battery24voltage"=0.0, "ErrorOutData"={"ErrorCode"=0, "ErrorMessage"=""}}, {"battery1voltage"=3.4816375, "battery2voltage"=3.4830372, "battery3voltage"=3.4783695, "battery4voltage"=3.482367, "battery5voltage"=3.4844053, "battery6voltage"=0.0, "battery7voltage"=0.0, "battery8voltage"=0.0, "battery9voltage"=0.0, "battery10voltage"=0.0, "battery11voltage"=0.0, "battery12voltage"=0.0, "battery13voltage"=0.0, "battery14voltage"=0.0, "battery15voltage"=0.0, "battery16voltage"=0.0, "battery17voltage"=0.0, "battery18voltage"=0.0, "battery19voltage"=0.0, "battery20voltage"=0.0, "battery21voltage"=0.0, "battery22voltage"=0.0, "battery23voltage"=0.0, "battery24voltage"=0.0, "ErrorOutData"={"ErrorCode"=0, "ErrorMessage"=""}}, {"battery1voltage"=3.4816375, "battery2voltage"=3.483041, "battery3voltage"=3.4783754, "battery4voltage"=3.4823663, "battery5voltage"=3.4843974, "battery6voltage"=0.0, "battery7voltage"=0.0, "battery8voltage"=0.0, "battery9voltage"=0.0, "battery10voltage"=0.0, "battery11voltage"=0.0, "battery12voltage"=0.0, "battery13voltage"=0.0, "battery14voltage"=0.0, "battery15voltage"=0.0, "battery16voltage"=0.0, "battery17voltage"=0.0, "battery18voltage"=0.0, "battery19voltage"=0.0, "battery20voltage"=0.0, "battery21voltage"=0.0, "battery22voltage"=0.0, "battery23voltage"=0.0, "battery24voltage"=0.0, "ErrorOutData"={"ErrorCode"=0, "ErrorMessage"=""}}, {"battery1voltage"=3.4816418, "battery2voltage"=3.4830368, "battery3voltage"=3.4783688, "battery4voltage"=3.4823596, "battery5voltage"=3.484408, "battery6voltage"=0.0, "battery7voltage"=0.0, "battery8voltage"=0.0, "battery9voltage"=0.0, "battery10voltage"=0.0, "battery11voltage"=0.0, "battery12voltage"=0.0, "battery13voltage"=0.0, "battery14voltage"=0.0, "battery15voltage"=0.0, "battery16voltage"=0.0, "battery17voltage"=0.0, "battery18voltage"=0.0, "battery19voltage"=0.0, "battery20voltage"=0.0, "battery21voltage"=0.0, "battery22voltage"=0.0, "battery23voltage"=0.0, "battery24voltage"=0.0, "ErrorOutData"={"ErrorCode"=0, "ErrorMessage"=""}}, {"battery1voltage"=3.4816406, "battery2voltage"=3.4830463, "battery3voltage"=3.4783697, "battery4voltage"=3.4823644, "battery5voltage"=3.484399, "battery6voltage"=0.0, "battery7voltage"=0.0, "battery8voltage"=0.0, "battery9voltage"=0.0, "battery10voltage"=0.0, "battery11voltage"=0.0, "battery12voltage"=0.0, "battery13voltage"=0.0, "battery14voltage"=0.0, "battery15voltage"=0.0, "battery16voltage"=0.0, "battery17voltage"=0.0, "battery18voltage"=0.0, "battery19voltage"=0.0, "battery20voltage"=0.0, "battery21voltage"=0.0, "battery22voltage"=0.0, "battery23voltage"=0.0, "battery24voltage"=0.0, "ErrorOutData"={"ErrorCode"=0, "ErrorMessage"=""}}, {"battery1voltage"=3.4816408, "battery2voltage"=3.4830425, "battery3voltage"=3.4783728, "battery4voltage"=3.4823697, "battery5voltage"=3.484402, "battery6voltage"=0.0, "battery7voltage"=0.0, "battery8voltage"=0.0, "battery9voltage"=0.0, "battery10voltage"=0.0, "battery11voltage"=0.0, "battery12voltage"=0.0, "battery13voltage"=0.0, "battery14voltage"=0.0, "battery15voltage"=0.0, 
